vi "MultiAxisMove.vi"(8 "error in (no error)":errorcluster, 11 "MotorController in":refnum<class "MotorController.lvclass">) -> (0 "error out":errorcluster, 3 "MotorController out":refnum<class "MotorController.lvclass">)   [LabVIEW 2019, in "MotorController.lvclass"]
uses:
  MotorController.lvclass
  MotorController.lvclass/MotorController.ctl
panel:
  in  "Stage Position":u16
  in  "Sample Position":u16
  in  "Polarizer 2 Position":u16
  in  "Polarizer 1 Position":u16
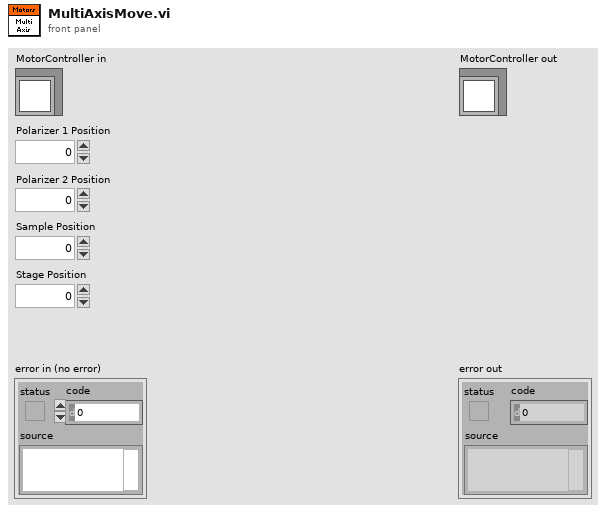
[diagram p1: front panel]
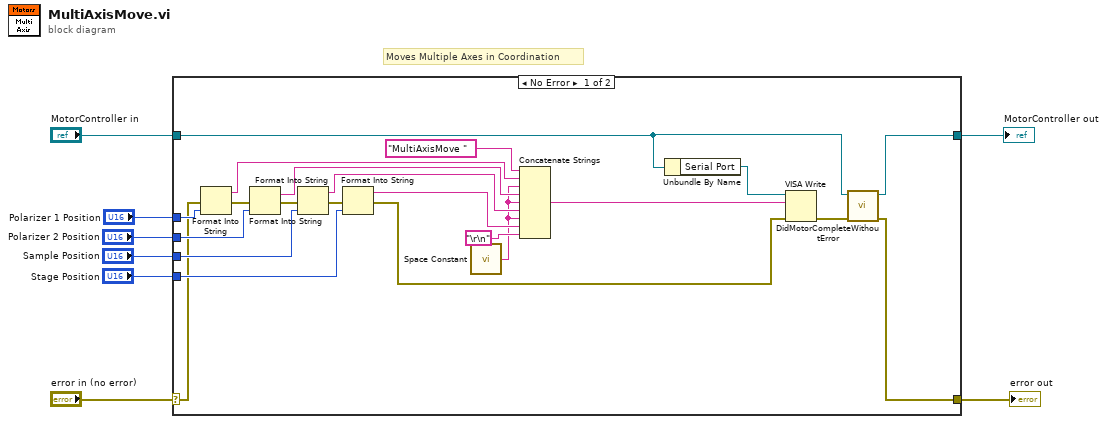
[diagram p0: block diagram]
diagram:
  # "Moves Multiple Axes in Coordination"
  n1 = case shown="No Error" "error in (no error)" {
    selector: "error in (no error)" -> [w23 w32]
    tunnel: [w11 w32] -> w7
    tunnel: [w13 w31] -> w5
    tunnel: "MotorController in" -> [w10 w31]
    tunnel: "Polarizer 1 Position" -> [w27 _]
    tunnel: "Polarizer 2 Position" -> [w26 _]
    tunnel: "Sample Position" -> [w25 _]
    tunnel: "Stage Position" -> [w24 _]
    frame No Error {
      n2 = Format Into String(error in=w23, w27) -> (resulting string=w21:string, error out=w30:errorcluster)  [unwired: 2 in]
      n3 = Format Into String(error in=w30, w26) -> (resulting string=w20:string, error out=w29:errorcluster)  [unwired: 2 in]
      n4 = Format Into String(error in=w29, w25) -> (resulting string=w19:string, error out=w28:errorcluster)  [unwired: 2 in]
      n5 = Format Into String(error in=w28, w24) -> (resulting string=w18:string, error out=w14:errorcluster)  [unwired: 2 in]
      n6 = call <vilib>:"Space Constant.vi"() -> ("String"=w16:string)
      n7 = Concatenate Strings("MultiAxisMove ", w21, w16, w20, w16, w19, w16, w18, "\r\n") -> (w15:string)
      n8 = Unbundle By Name(w10) -> ("Serial Port"=w9:refnum<visa-resource-name>)
      n9 = VISA Write(VISA resource name=w9, write buffer=w15, error in (no error)=w14) -> (error out=w12:errorcluster)  [unwired: 2 out]
      n10 = call "DidMotorCompleteWithoutError.vi"("error in (no error)"=w12, "MotorController in"=w10) -> ("error out"=w11:errorcluster, "MotorController out"=w13:refnum<class "MotorController.lvclass">)  [unwired: 7 in, 1 out]
    }
    frame Error {
    }
  }
  "error out" <- w7
  "MotorController out" <- w5
